vi "Results (2D) to X and Y Arrays.vi"(11 "Results":dbl[][](array[numeric])) -> (2 "Y":dbl[](array[numeric]), 3 "X":dbl[](array[numeric]))   [LabVIEW 2016, in "Transport.lvclass"]
uses:
  Transport.lvclass
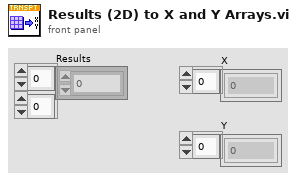
[diagram p1: front panel]
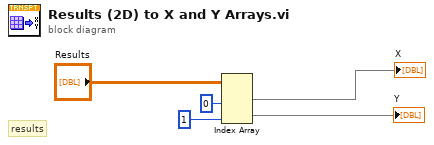
[diagram p0: block diagram]
diagram:
  # "results"
  n1 = Index Array(array="Results", index (col) #1=0 ("disabled index (col)"), index (col) #2=1 ("index (col)")) -> (element #1=→"X":dbl[], element #2=→"Y":dbl[])  [unwired: 2 in]
